vi "Keithley 2002 Read Query.vi"(7 "function (Vdc:1)":u16(ring)=1 items=["ac voltage", "dc voltage", "2-wire resistance", "4-wire resistance", "ac current", "dc current", "frequency", "temperature"], 8 "error in":T1, 10 "timeout ms":u32=10000, 11 "GPIB Address":string) -> (0 "error out":T1, 3 "Reading Result":string)   [LabVIEW 2020]
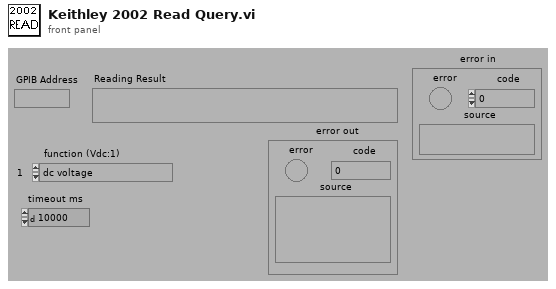
[diagram p1: front panel]
types:
  T1 = cluster{"error":bool, "code":i32, "source":string}
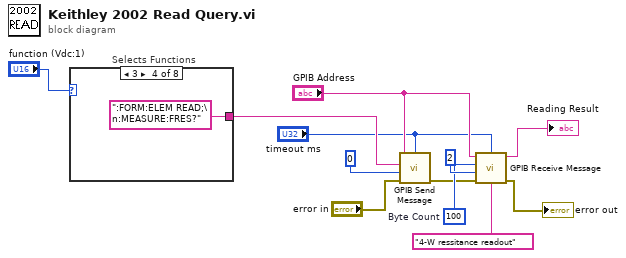
[diagram p0: block diagram]
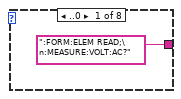
[diagram p2: hidden frame]
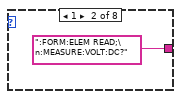
[diagram p3: hidden frame]
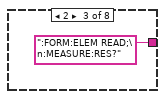
[diagram p4: hidden frame]
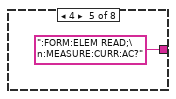
[diagram p5: hidden frame]
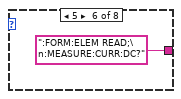
[diagram p6: hidden frame]
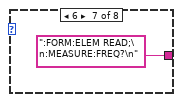
[diagram p7: hidden frame]
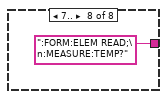
[diagram p8: hidden frame]
diagram:
  w9 = 100  # Byte Count
  n1 = case "Selects Functions" shown="3" "function (Vdc:1)" {
    tunnel: [":FORM:ELEM READ;\n:MEASURE:VOLT:AC?" ":FORM:ELEM READ;\n:MEASURE:VOLT:DC?" ":FORM:ELEM READ;\n:MEASURE:RES?" ":FORM:ELEM READ;\n:MEASURE:FRES?" ":FORM:ELEM READ;\n:MEASURE:CURR:AC?" ":FORM:ELEM READ;\n:MEASURE:CURR:DC?" ":FORM:ELEM READ;\n:MEASURE:FREQ?\n" ":FORM:ELEM READ;\n:MEASURE:TEMP?"] -> w3
    frame ..0 {
    }
    frame 1 {
    }
    frame 2 {
    }
    frame 3 {
    }
    frame 4 {
    }
    frame 5 {
    }
    frame 6 {
    }
    frame 7.. {
    }
  }
  n2 = call "GPIB Send Message.vi"("timeout ms"="timeout ms", "address string"="GPIB Address", "write buffer"=w3, "write mode (set END:0)"=0, "error in"="error in") -> ("error out"=w6:T1)  [unwired: 2 in, 2 out]
  n3 = call "GPIB Receive Message.vi"("timeout ms"="timeout ms", "address string"="GPIB Address", "byte count"=w9, "source"="4-W ressitance readout", "read mode"=2, "error in"=w6) -> ("read buffer"=→"Reading Result":string, "error out"=→"error out":T1)  [unwired: 1 in, 1 out]
